vi "KHFAC and Amplitude Generation V3.vi"() -> ()   [LabVIEW 2020]
uses:
  <vilib>/measure/NI_MAPro.lvlib
  <vilib>/measure/NI_MABase.lvlib
panel:
  in  "Waveform Type":u16(ring) items=["Sine Wave", "Triangle Wave", "Square Wave", "Sawtooth Wave"]
  out "Waveform Graph":waveform(dbl)[](graph)
  in  "Step Length (s)":i64
  in  "Step Size (Vpp)":dbl
  in  "Initial Step Length (s)":i64
  in  "End Voltage (Vpp)":dbl
  in  "Initial Voltage (Vpp)":dbl
  out "Sampling Frequency":dbl
  in  "Samples/Cycle":dbl
  in  "Waveform Frequency":dbl
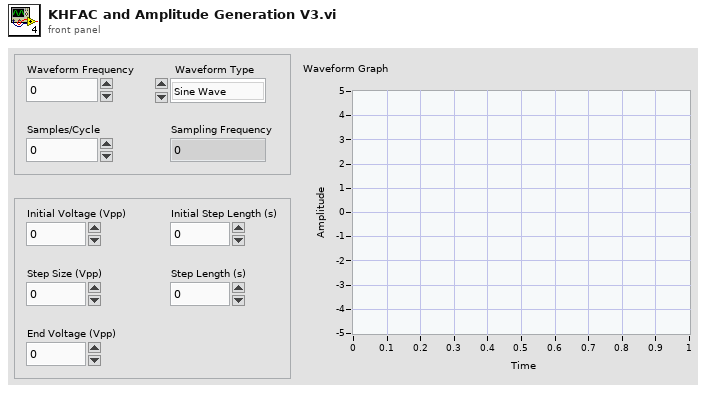
[diagram p1: front panel]
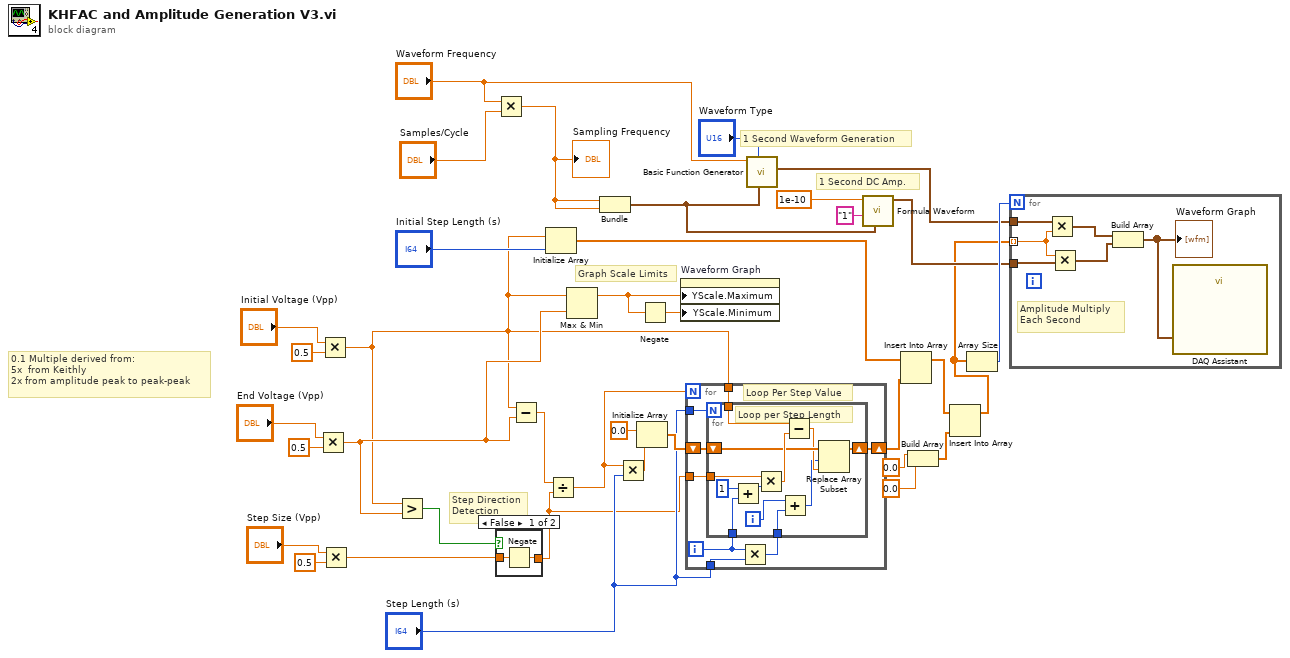
[diagram p0: block diagram]
diagram:
  # "Graph Scale Limits"
  # "Step Direction\nDetection"
  # "0.1 Multiple derived from:\n5x  from Keithly\n2x from amplitude peak to peak-peak"
  # "1 Second DC Amp."
  # "1 Second Waveform Generation"
  n1 = Multiply(x="End Voltage (Vpp)", y=0.5) -> (x*y=w2:dbl)
  n2 = Multiply(x="Initial Voltage (Vpp)", y=0.5) -> (x*y=w1:dbl)
  n3 = Multiply(x="Step Size (Vpp)", y=0.5) -> (x*y=w9:dbl)
  n4 = Greater?(x=w1, y=w2) -> (0:w4:bool)
  n5 = Multiply(x="Waveform Frequency", y="Samples/Cycle") -> (x*y=w31:dbl)
  "Sampling Frequency" <- w31
  n6 = case shown="False" w4 {
    tunnel: w9 -> [w39 w40]
    tunnel: [w38 w40] -> w8
    frame False {
      n7 = Negate(x=w39) -> (-x=w38:dbl)
    }
    frame True {
    }
  }
  n8 = Subtract(x=w1, y=w2) -> (x-y=w36:dbl)
  n9 = Initialize Array(w1, "Initial Step Length (s)") -> (w28:dbl[])
  n10 = Divide(x=w36, y=w8) -> (x/y=w24:dbl)
  n11 = Max & Min(x=w1, y=w2) -> (max(x,y)=w3:dbl)  [unwired: 1 out]
  n12 = Bundle(w31, w31) -> (w14:cluster{dbl, dbl})  [unwired: 1 in]
  n13 = Multiply(x=w24, y="Step Length (s)") -> (x*y=w25:dbl)
  n14 = Initialize Array(0.0 ("element"), w25) -> (w29:dbl[])
  n15 = Negate(x=w3) -> (-x=w11:dbl)
  n16 = property on="Waveform Graph" class="WFGraph (strict)"("YScale.Maximum"=w3, "YScale.Minimum"=w11) -> ()  [unwired: 2 in, 2 out]
  n17 = for {
    N: w24 -> [_]
    tunnel: w8 -> [w48]
    tunnel: w1 -> [w47]
    shift-right: [w45] -> w27
    shift-left: w29 -> [w46]
    tunnel: "Step Length (s)" -> [w44]
    tunnel: "Step Length (s)" -> [w42]
    i -> [w41]
    # "Loop Per Step Value"
    n18 = Multiply(x=w41, y=w42) -> (x*y=w43:i64)
    n19 = for {
      N: w44 -> [_]
      tunnel: w48 -> [w60]
      tunnel: w47 -> [w58]
      tunnel: w43 -> [w50]
      shift-right: [w55] -> w45
      shift-left: w46 -> [w57]
      tunnel: w41 -> [w49]
      i -> [w51]
      # "Loop per Step Length"
      n20 = Add(x=1, y=w49) -> (x+y=w53:i32)
      n21 = Multiply(x=w60, y=w53) -> (x*y=w59:dbl)
      n22 = Add(x=w51, y=w50) -> (x+y=w52:i64)
      n23 = Subtract(x=w58, y=w59) -> (x-y=w56:dbl)
      n24 = Replace Array Subset(array=w57, new element=w56, index=w52) -> (w55:dbl[])
    }
  }
  n25 = call <vilib>:"Basic Function Generator.vi"("sampling info"=w14, "signal type"="Waveform Type", "frequency"="Waveform Frequency") -> ("signal out"=w15:waveform(dbl))  [unwired: 6 in, 2 out]
  n26 = call <vilib>:"Formula Waveform.vi"("sampling info"=w14, "formula"="1", "frequency"=1e-10) -> ("signal out"=w21:waveform(dbl))  [unwired: 7 in, 1 out]
  n27 = Insert Into Array(array=w28, new element=w27) -> (w20:dbl[])  [unwired: 1 in]
  n28 = Build Array(0.0 ("element"), 0.0 ("element")) -> (w18:dbl[])
  n29 = Insert Into Array(array=w20, new element=w18) -> (w19:dbl[])  [unwired: 1 in]
  n30 = Array Size(array=w19) -> (size(s)=w26:i32)
  n31 = for {
    N: w26 -> [_]
    tunnel: w19 -> [w62] mode=indexing
    tunnel: w15 -> [w66]
    tunnel: w21 -> [w63]
    # "Amplitude Multiply\nEach Second"
    n32 = Multiply(x=w66, y=w62) -> (x*y=w65:waveform(dbl))
    n33 = Multiply(x=w62, y=w63) -> (x*y=w64:waveform(dbl))
    n34 = Build Array(w65, w64) -> (w61:waveform(dbl)[])
    "Waveform Graph" <- w61
    n35 = call "DAQ Assistant"("data"=w61) -> ()  [unwired: 16 in, 3 out]
  }
